vi "Cálculos.vi"(2 "Dados in":T2, 3 "IP":T1={"Diâmetro do furo [mm]"=1.4, "Diâmetro da linha média [mm]"=5.0, "IncF"=0.2, "Módulo de elasticidade [GPa]"=207.0, "Módulo de Poisson"=0.3, "Tipo de roseta utilizada"=enum."Tipo A", "Método de análise"=enum."Simplificado 2008", "Pfinal"=0.3, "Parar auto."=TRUE} caption="Infos para processamento") -> (0 "Círculo de Mohr":cluster{"Array":dbl[], "Array":dbl[]}[][](array[cluster]), 1 "Resultados":dbl[][](array[numeric]))   [LabVIEW 2016]
uses:
  Controles/p,q, t, a e b.ctl
  Controles/Infos para processamento.ctl
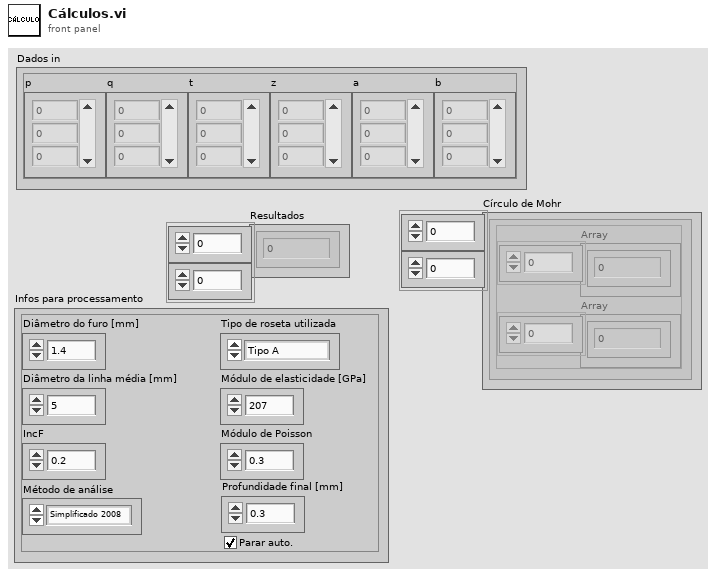
[diagram p1: front panel]
types:
  T1 = typedef "Infos para processamento.ctl" = cluster{"Diâmetro do furo [mm]":dbl, "Diâmetro da linha média [mm]":dbl, "IncF":dbl, "Módulo de elasticidade [GPa]":dbl, "Módulo de Poisson":dbl, "Tipo de roseta utilizada":enum16{"Tipo A", "Tipo B", "Tipo C"}, "Método de análise":enum16{"Não uniforme 2013", "Simplificado 2013", "Simplificado 2008"}, "Pfinal":dbl, "Parar auto.":bool}
  T2 = typedef "p,q, t, a e b.ctl" = cluster{"p":dbl[], "q":dbl[], "t":dbl[], "z":dbl[], "a":dbl[], "b":dbl[]}
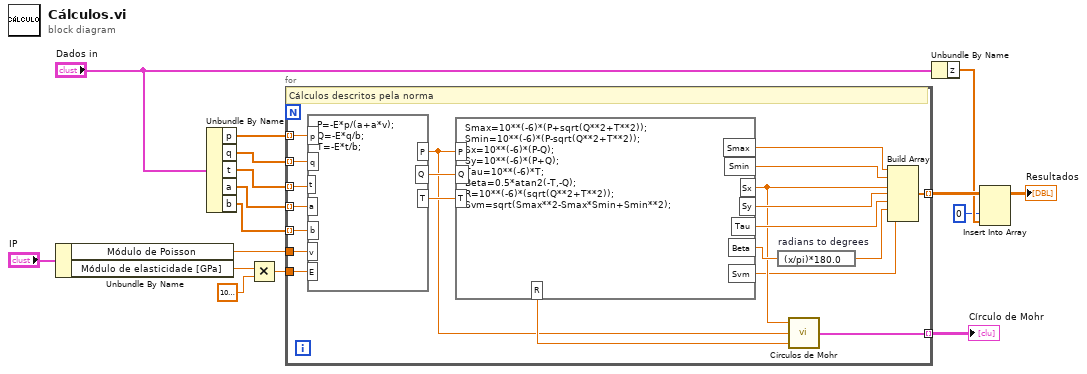
[diagram p0: block diagram]
diagram:
  n1 = Unbundle By Name("IP") -> ("Módulo de Poisson"=w2:dbl, "Módulo de elasticidade [GPa]"=w1:dbl)
  n2 = Unbundle By Name("Dados in") -> ("p"=w11:dbl[], "q"=w12:dbl[], "t"=w13:dbl[], "a"=w14:dbl[], "b"=w15:dbl[])
  n3 = Multiply(x=w1, y=1000000000.0) -> (x*y=w3:dbl)
  n4 = for {
    tunnel: w11 -> [w37] mode=indexing
    tunnel: w12 -> [w36] mode=indexing
    tunnel: w13 -> [w35] mode=indexing
    tunnel: w3 -> [w34]
    tunnel: w2 -> [w33]
    tunnel: w14 -> [w32] mode=indexing
    tunnel: w15 -> [w31] mode=indexing
    tunnel: [w28] -> w9 mode=indexing
    tunnel: [w18] -> w16 mode=indexing
    # "Cálculos descritos pela norma"
    n5 = formula code="P=-E*p/(a+a*v);\nQ=-E*q/b;\nT=-E*t/b;"("p"=w37, "q"=w36, "t"=w35, "E"=w34, "v"=w33, "a"=w32, "b"=w31) -> ("P"=w19:dbl, "Q"=w25:dbl, "T"=w24:dbl)
    n6 = formula code="Smax=10**(-6)*(P+sqrt(Q**2+T**2));\nSmin=10**(-6)*(P-sqrt(Q**2+T**2));\nSx=10**(-6)*(P-Q);\nSy=10**(-6)*(P+Q);\nTau=10**(-6)*T;\nBeta=0.5*atan2(-T,-Q);\nR=10**(-6)*(sqrt(Q**2+T**2));\nSvm=sqrt(Smax**2-Smax*Smin+Smin**2);"("P"=w19, "Q"=w25, "T"=w24) -> ("Smax"=w27:dbl, "Smin"=w26:dbl, "Sx"=w21:dbl, "Sy"=w30:dbl, "Tau"=w29:dbl, "Beta"=w23:dbl, "R"=w20:dbl, "Svm"=w17:dbl)
    n7 = expression code="(x/pi)*180.0" "radians to degrees"(w23) -> (w22:dbl)
    n8 = call "Círculos de Mohr.vi"("R"=w20, "P"=w19, "Sx"=w21) -> ("Círculo de Mohr"=w18:cluster{"Array":dbl[], "Array":dbl[]}[])
    n9 = Build Array(w27, w26, w21, w30, w29, w22, w17) -> (w28:dbl[])
  }
  "Círculo de Mohr" <- w16
  n10 = Unbundle By Name("Dados in") -> ("z"=w8:dbl[])
  n11 = Insert Into Array(array=w9, index (col)=0 ("disabled index (col)"), new element=w8) -> (→"Resultados":dbl[][])  [unwired: 1 in]
